vi "FindMinimumChiSquaredFast.vi"(2 "Restrict to Positive Imaginary Part":bool=TRUE, 3 "Starting points 2":dbl[][](array[numeric])=[[1.5, 0.1], [1.5, 0.11], [1.52, 0.1]], 4 "Simplex Graph":refnum<vi>, 5 "Extinction ExtinctionUncertainity Size parameter and Number ofS sizes":T1={"PAS amplitude"=[], "PAS amp Uncertainty"=[], "Size parameters"=[], "Number ofSizes"=0.0, "GeometricCrossSection"=[], "Wave Length"=0.0, "SMPS Sizes"=[], "Concentration"=[], "Double Charge Correction"=FALSE, "Extincation Factor"=1.0, "Diameter Factor"=1.0, "Diameter Offset"=0.0, "Extinction Factor Flag"=FALSE, "Diameter Factor Flag"=FALSE, "Diameter Offset Flag"=FALSE, "Sizes"=[], "ExtinctionOrAbsorptionOrScattering"=0, "Concentration(#/cc)"=[]} {"ExtinctionOrAbsorptionOrScattering" scale=0.0..2.0}) -> (0 "Imaginary Part from fit":dbl=0.051495699826118665, 1 "Real Part from fit":dbl=1.57799797397569)   [LabVIEW 2013]
uses:
  BaesDataTypeDefinition.ctl
  RTDownhillSimplex.llb/RTDownhillSimplexGlobals.vi
panel:
  in  "Convergence Strength":dbl=1e-05
  out "Waveform Chart":i32(graph)=60
  out "Starting points 3":dbl[][](array[numeric])=[[1.6630594557043747, 0.246532961950036], [1.4605000230939145, 0.15705446819563057], [1.5705619064033547, 0.05175990620612842]]
  in  "Downhill-Simplex parameters 2":T2={"alpha"=1.0, "beta"=0.5, "gamma"=2.0, "Maximum"=FALSE}
  out "Stopping condition flag":bool=TRUE
  out "x-y":dbl[](array[numeric])=[0.000168992022227199, 0.00018933075538369454]
  in  "buzzer":bool
  in  "Continous":bool=TRUE
  in  "sleep-time":dbl
  out "Simplex":cluster{dbl[], dbl[]}[](graph)=[{[1.57799797397569, 1.5778289819534628, 1.5778839622345557, 1.57799797397569], [0.051495699826118665, 0.05130636907073497, 0.05144020076942982, 0.051495699826118665]}]
  out "ValueInput":dbl=0.9201608571739257 format="%#_8g"
  out "ValueOutput":dbl=0.920166987183041 format="%#_8g"
  out "newSimplexPoint":dbl[](array[numeric])=[1.57799797397569, 0.051495699826118665]
  in  "Testfunction":enum16{"Rosenbrock function", "PID Controller"}(ring)=enum."PID Controller"
  in  "Downhill-Simplex parameters":T2={"alpha"=1.0, "beta"=0.5, "gamma"=2.0, "Maximum"=FALSE}
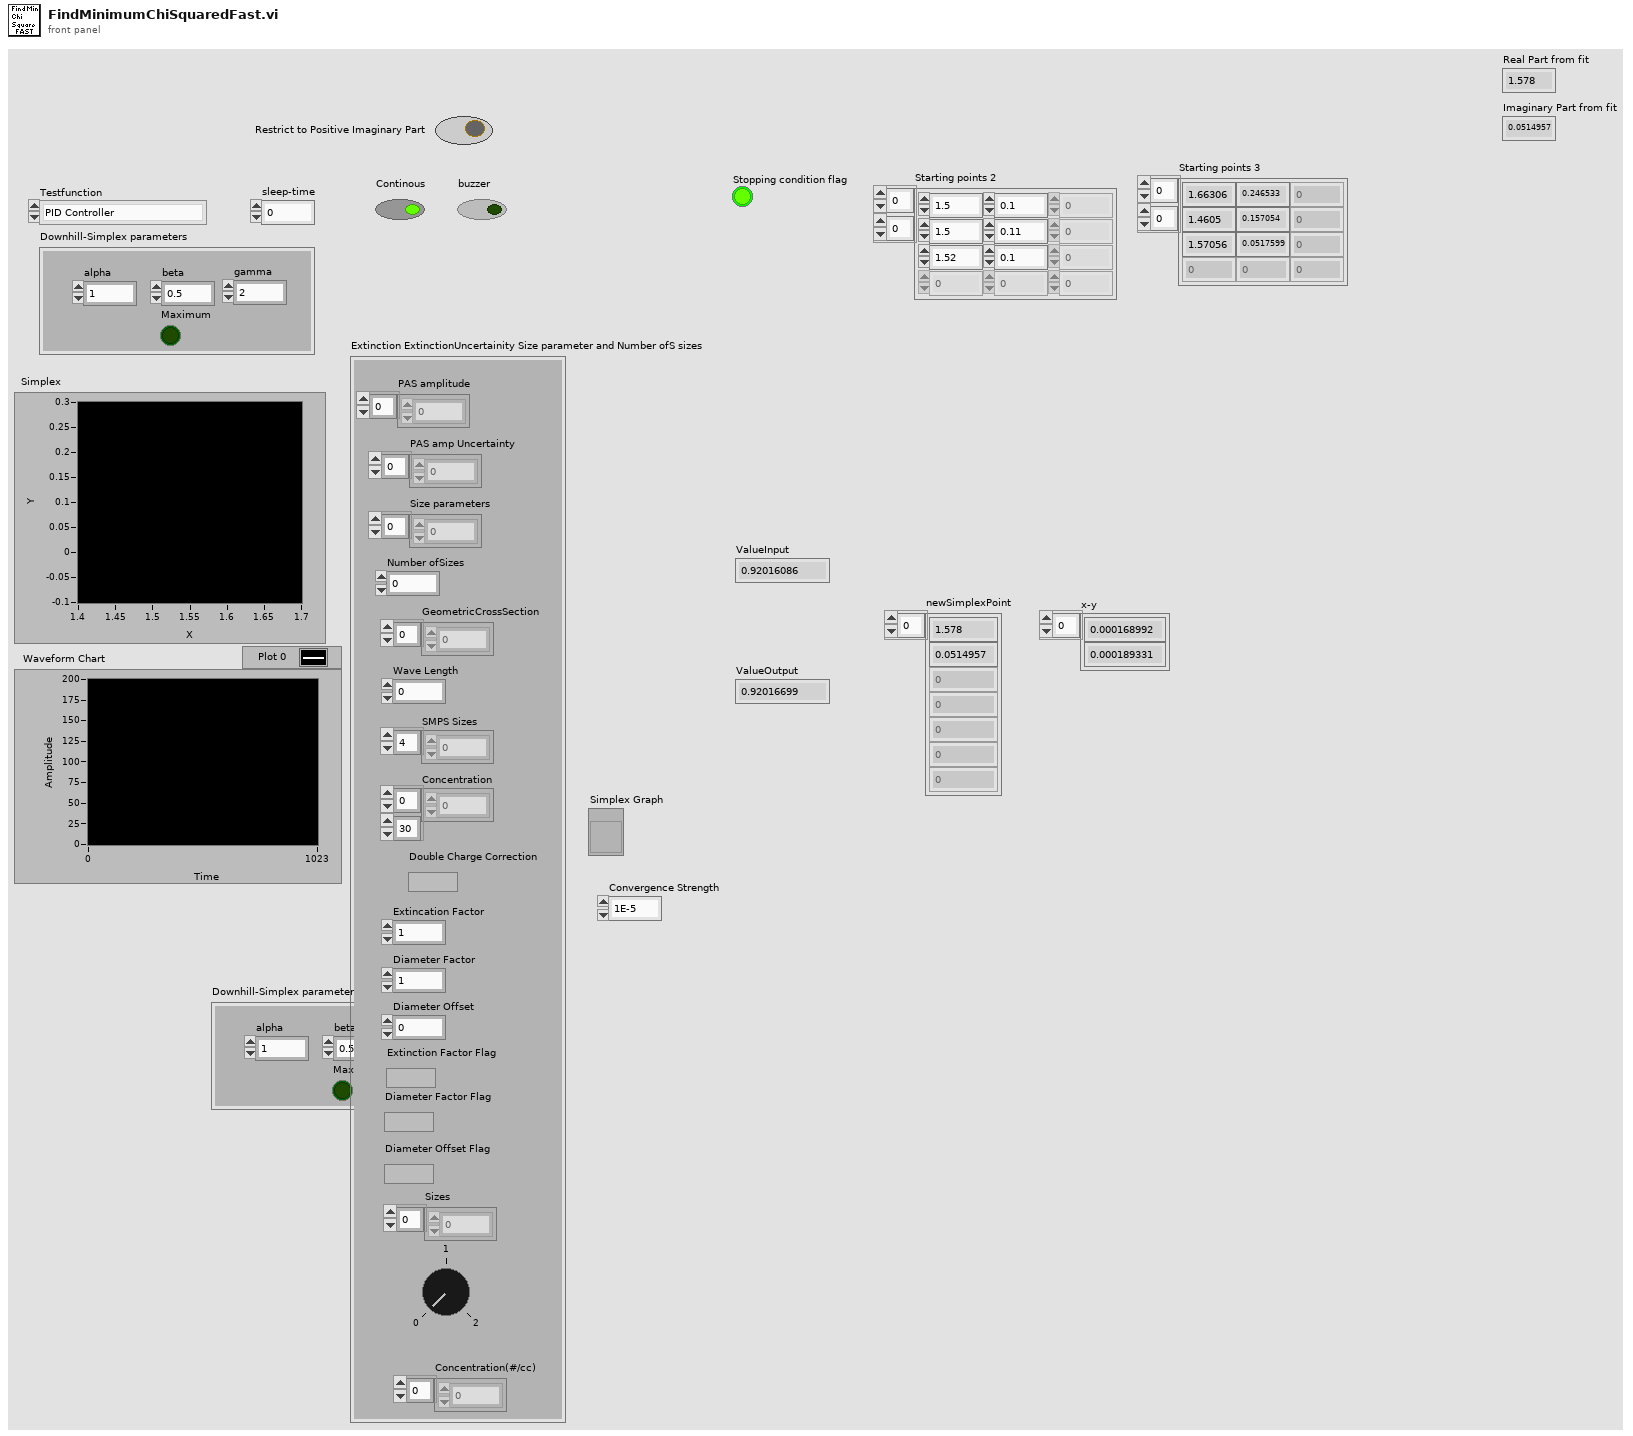
[diagram p1: front panel]
types:
  T1 = typedef "BaesDataTypeDefinition.ctl" = cluster{"PAS amplitude":dbl[], "PAS amp Uncertainty":dbl[], "Size parameters":dbl[], "Number ofSizes":dbl, "GeometricCrossSection":dbl[], "Wave Length":dbl, "SMPS Sizes":dbl[], "Concentration":dbl[][], "Double Charge Correction":bool, "Extincation Factor":dbl, "Diameter Factor":dbl, "Diameter Offset":dbl, "Extinction Factor Flag":bool, "Diameter Factor Flag":bool, "Diameter Offset Flag":bool, "Sizes":dbl[], "ExtinctionOrAbsorptionOrScattering":i8, "Concentration(#/cc)":dbl[]}
  T2 = cluster{"alpha":dbl, "beta":dbl, "gamma":dbl, "Maximum":bool}
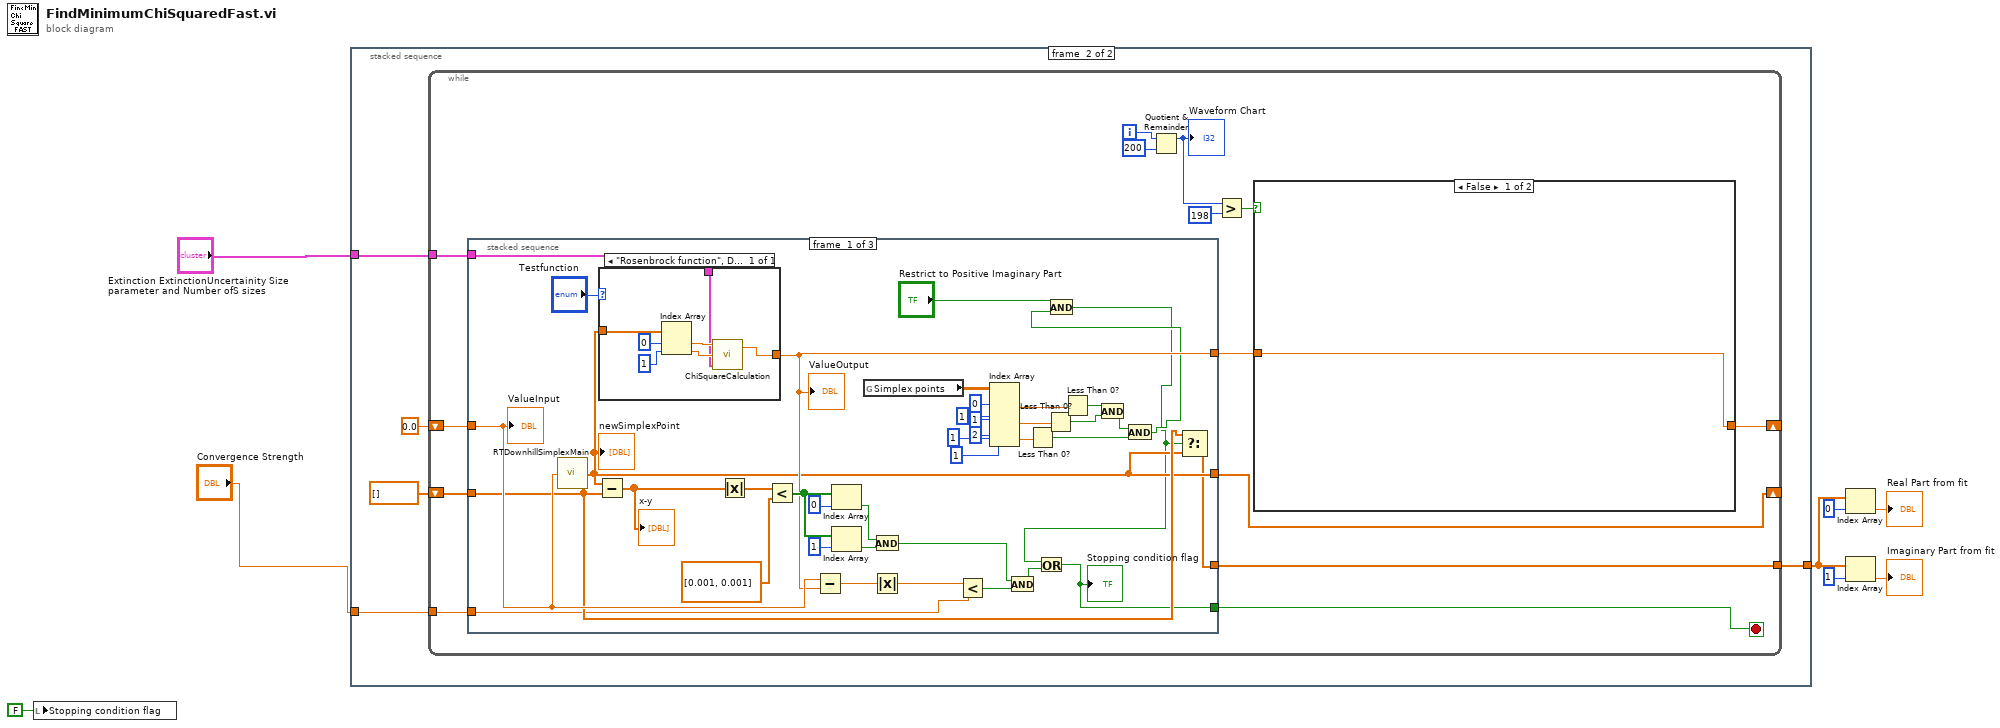
[diagram p0: block diagram]
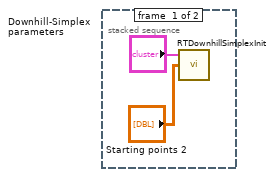
[diagram p2: hidden frame]
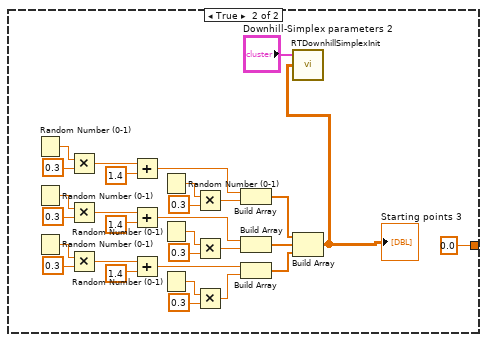
[diagram p3: hidden frame]
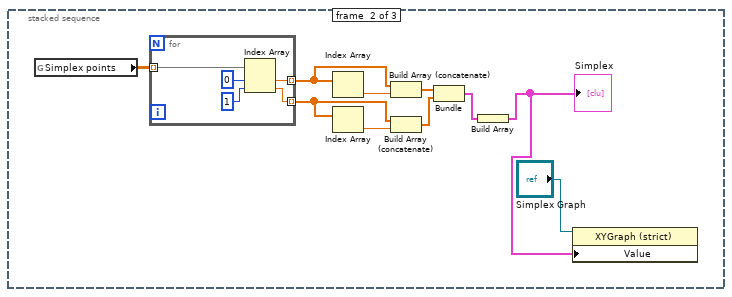
[diagram p4: hidden frame]
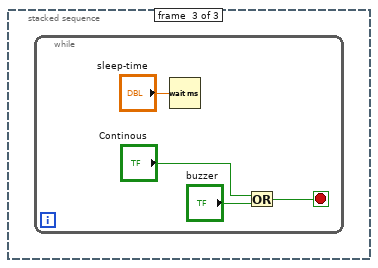
[diagram p5: hidden frame]
diagram:
  n1 = local write "Stopping condition flag"(FALSE ("Stopping condition flag")) -> ()
  n2 = stacked-sequence {
    tunnel: [_ w13] -> w5
    tunnel: "Extinction ExtinctionUncertainity Size parameter and Number ofS sizes" -> [_ w12]
    tunnel: "Convergence Strength" -> [_ w11]
    frame #0 {
      n3 = call "RTDownhillSimplexInit.vi"("Starting points"="Starting points 2", "Downhill-Simplex parameters"="Downhill-Simplex parameters") -> ()  [unwired: 2 in]
    }
    frame #1 {
      n4 = while {
        shift-right: [w22] -> _
        shift-left: 0.0 -> [w29]
        shift-right: [w28] -> _
        shift-left: dbl[] [] ("newSimplexPoint") -> [w27]
        tunnel: [w26] -> w13
        tunnel: w12 -> [w18]
        tunnel: w11 -> [w16]
        i -> [w21]
        stop <- w17 stop-if-true
        n5 = stacked-sequence {
          tunnel: w29 -> [w89 _ _]
          tunnel: [w88 _ _] -> w23
          tunnel: [w67 _ _] -> w28
          tunnel: w27 -> [w68 _ _]
          tunnel: [w66 _ _] -> w26
          tunnel: w18 -> [w84 _ _]
          tunnel: [w65 _ _] -> w17
          tunnel: w16 -> [w61 _ _]
          frame #0 {
            n6 = call "RTDownhillSimplexMain.vi"("newSimplexValue"=w89) -> ("newSimplexPoint"=w67:dbl[])
            "newSimplexPoint" <- w67
            n7 = Subtract(x=w67, y=w68) -> (x-y=w98:dbl[])
            "x-y" <- w98
            n8 = case shown="\"Rosenbrock function\", Default" "Testfunction" {
              tunnel: w67 -> [w106]
              tunnel: [w101] -> w88
              tunnel: w84 -> [w100]
              frame "Rosenbrock function", Default {
                n9 = Index Array(array=w106, index #1=0 ("index"), index #2=1 ("index")) -> (element #1=w103:dbl, element #2=w102:dbl)
                n10 = call "ChiSquareCalculation.vi"("Extinction ExtinctionUncertainity Size parameter and Number ofS sizes 2"=w100, "refractive index, imaginary"=w102, "refractive index, real"=w103) -> ("Chi Squared"=w101:dbl)  [unwired: 1 out]
              }
            }
            "ValueOutput" <- w88
            n11 = Absolute Value(x=w98) -> (abs(x)=w97:dbl[])
            n12 = Less?(x=w97, y=dbl[] [0.001, 0.001]) -> (x < y?=w93:bool[])
            n13 = Subtract(x=w89, y=w88) -> (x-y=w90:dbl)
            n14 = Index Array(array=w93, index=0) -> (element=w92:bool)
            n15 = Index Array(array=w93, index=1) -> (element=w91:bool)
            n16 = global read "RTDownhillSimplexGlobals.vi" "Simplex points"() -> (w82:dbl[][])
            n17 = And(x=w92, y=w91) -> (x .and. y?=w86:bool)
            n18 = Absolute Value(x=w90) -> (abs(x)=w87:dbl)
            n19 = Less?(x=w87, y=w61) -> (x < y?=w85:bool)
            n20 = Index Array(array=w82, index (row) #1=0 ("index (row)"), index (col) #1=1 ("disabled index (col)"), index (row) #2=1 ("index (row)"), index (col) #2=1 ("disabled index (col)"), index (row) #3=2 ("index (row)"), index (col) #3=1 ("disabled index (col)")) -> (element #1=w75:dbl, element #2=w74:dbl, element #3=w73:dbl)
            n21 = And(x=w86, y=w85) -> (x .and. y?=w83:bool)
            n22 = Less Than 0?(x=w73) -> (x < 0?=w69:bool)
            n23 = Less Than 0?(x=w74) -> (x < 0?=w71:bool)
            n24 = Less Than 0?(x=w75) -> (x < 0?=w72:bool)
            n25 = And(x=w72, y=w71) -> (x .and. y?=w70:bool)
            n26 = And(x=w70, y=w69) -> (x .and. y?=w63:bool)
            n27 = And(x="Restrict to Positive Imaginary Part", y=w63) -> (x .and. y?=w62:bool)
            n28 = Or(x=w62, y=w83) -> (x .or. y?=w65:bool)
            "Stopping condition flag" <- w65
            n29 = Select(t=w68, s=w62, f=w67) -> (s? t:f=w66:dbl[])
            "ValueInput" <- w89
          }
          frame #1 {
            n30 = global read "RTDownhillSimplexGlobals.vi" "Simplex points"() -> (w110:dbl[][])
            n31 = for {
              tunnel: w110 -> [w121] mode=indexing
              tunnel: [w118] -> w115 mode=indexing
              tunnel: [w117] -> w112 mode=indexing
              n32 = Index Array(array=w121, index #1=0 ("index"), index #2=1 ("index")) -> (element #1=w118:dbl, element #2=w117:dbl)
            }
            n33 = Index Array(array=w115) -> (element=w116:dbl)  [unwired: 1 in]
            n34 = Index Array(array=w112) -> (element=w113:dbl)  [unwired: 1 in]
            n35 = Build Array (concatenate)(w115, w116) -> (w114:dbl[])
            n36 = Build Array (concatenate)(w112, w113) -> (w111:dbl[])
            n37 = Bundle(w114, w111) -> (w109:cluster{dbl[], dbl[]})  [unwired: 1 out]
            n38 = Build Array(w109) -> (w107:cluster{dbl[], dbl[]}[])
            "Simplex" <- w107
            n39 = property class="XYGraph (strict)"(reference="Simplex Graph", "Value"=w107) -> ()  [unwired: 1 in, 2 out]
          }
          frame #2 {
            n40 = while {
              stop <- w124 stop-if-true
              n41 = Wait (ms)(milliseconds to wait="sleep-time") -> ()  [unwired: 1 out]
              n42 = Or(x="Continous", y="buzzer") -> (x .or. y?=w124:bool)
            }
          }
        }
        n43 = Quotient & Remainder(x=w21, y=200) -> (x-y*floor(x/y)=w19:i32)  [unwired: 1 out]
        "Waveform Chart" <- w19
        n44 = Greater?(x=w19, y=198) -> (0:w24:bool)
        n45 = case shown="False" w24 {
          tunnel: [w30 0.0 ("Chi Squared")] -> w22
          tunnel: w23 -> [w30 _]
          frame False {
          }
          frame True {
            n46 = Random Number (0-1)() -> (number: 0 to 1=w49:dbl)
            n47 = Random Number (0-1)() -> (number: 0 to 1=w45:dbl)
            n48 = Random Number (0-1)() -> (number: 0 to 1=w41:dbl)
            n49 = Multiply(x=w49, y=0.3) -> (x*y=w47:dbl)
            n50 = Multiply(x=w45, y=0.3) -> (x*y=w43:dbl)
            n51 = Multiply(x=w41, y=0.3) -> (x*y=w39:dbl)
            n52 = Add(x=w47, y=1.4) -> (x+y=w37:dbl)
            n53 = Add(x=w43, y=1.4) -> (x+y=w35:dbl)
            n54 = Add(x=w39, y=1.4) -> (x+y=w33:dbl)
            n55 = Random Number (0-1)() -> (number: 0 to 1=w55:dbl)
            n56 = Random Number (0-1)() -> (number: 0 to 1=w53:dbl)
            n57 = Random Number (0-1)() -> (number: 0 to 1=w51:dbl)
            n58 = Multiply(x=w55, y=0.3) -> (x*y=w36:dbl)
            n59 = Multiply(x=w53, y=0.3) -> (x*y=w34:dbl)
            n60 = Multiply(x=w51, y=0.3) -> (x*y=w32:dbl)
            n61 = Build Array(w37, w36) -> (w58:dbl[])
            n62 = Build Array(w35, w34) -> (w57:dbl[])
            n63 = Build Array(w33, w32) -> (w56:dbl[])
            n64 = Build Array(w58, w57, w56) -> (w31:dbl[][])
            "Starting points 3" <- w31
            n65 = call "RTDownhillSimplexInit.vi"("Starting points"=w31, "Downhill-Simplex parameters"="Downhill-Simplex parameters 2") -> ()  [unwired: 2 in]
          }
        }
      }
    }
  }
  n66 = Index Array(array=w5, index=0) -> (element=→"Real Part from fit":dbl)
  n67 = Index Array(array=w5, index=1) -> (element=→"Imaginary Part from fit":dbl)
